vi "Calculator_sum-teardown.vi"(8 "test case ID":string, 10 "x+y":dbl, 11 "Calculator out":refnum<class "Calculator.lvclass">) -> (3 "result":bool)   [LabVIEW 2018]
doc: "The teardown VI should be executed after the VI under test in the harness VI. In this VI you can evaluate the outputs of the VI under test.\n\nSee the Help Document for more information. (<b>Help</b> > <b>InstaCoverage Help...</b>)"
uses:
  Calculator.lvclass
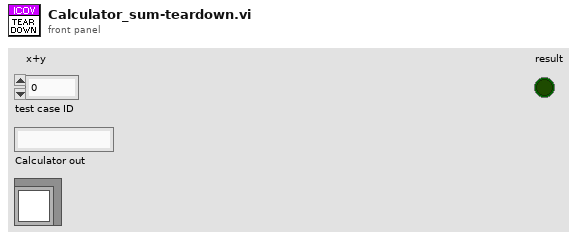
[diagram p1: front panel]
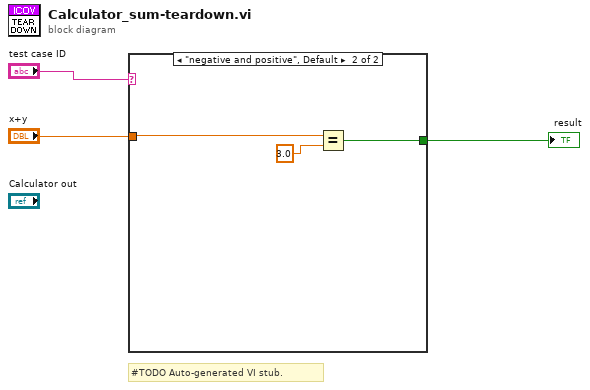
[diagram p0: block diagram]
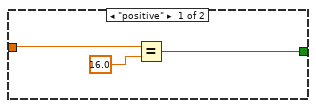
[diagram p2: hidden frame]
diagram:
  # "#TODO Auto-generated VI stub."
  n1 = case shown="\"negative and positive\", Default" "test case ID" {
    tunnel: [w4 w8] -> w2
    tunnel: "x+y" -> [w5 w7]
    frame "positive" {
      n2 = Equal?(x=w5, y=16.0) -> (x = y?=w4:bool)
    }
    frame "negative and positive", Default {
      n3 = Equal?(x=w7, y=3.0) -> (x = y?=w8:bool)
    }
  }
  "result" <- w2
